vi "Delete.vi"(8 "error in (no error)":errorcluster, 11 "Timer in":refnum<class "Timer.lvclass">) -> (0 "error out":errorcluster)   [LabVIEW 2020, in "Timer.lvclass"]
uses:
  Timer.lvclass
  Timer.lvclass/Timer.ctl
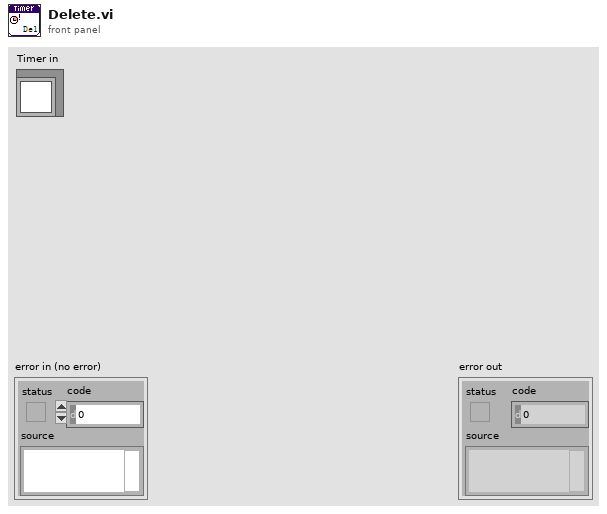
[diagram p1: front panel]
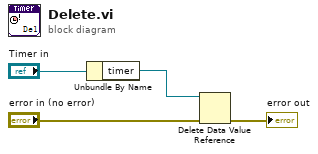
[diagram p0: block diagram]
diagram:
  n1 = Unbundle By Name("Timer in") -> ("timer"=w2:refnum<data-value>)
  n2 = Delete Data Value Reference(data value reference=w2, error in="error in (no error)") -> (error out=→"error out":errorcluster)  [unwired: 1 out]
